vi "FGVData.vi"(7 "Enum":T1, 8 "error in":errorcluster, 9 "DataIn":sgl[](array[numeric])) -> (0 "error out":errorcluster, 1 "DataOut":sgl[](array[numeric]))   [LabVIEW 2016]
uses:
  controls/Enum.ctl
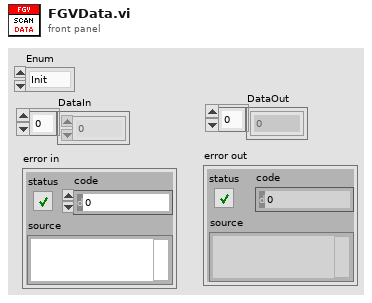
[diagram p1: front panel]
types:
  T1 = typedef "Enum.ctl" = enum16{"Init", "Read", "Write"}
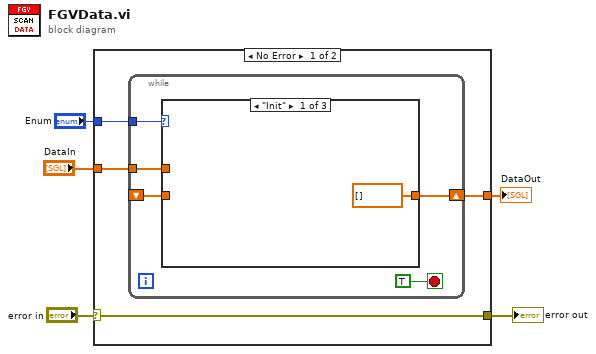
[diagram p0: block diagram]
diagram:
  n1 = case shown="No Error" "error in" {
    selector: "error in" -> [w8 w19]
    tunnel: "Enum" -> [w9 _]
    tunnel: [w8 w19] -> w4
    tunnel: "DataIn" -> [w7 w18]
    tunnel: [w6 w18] -> w1
    frame No Error {
      n2 = while {
        tunnel: w9 -> [w13]
        tunnel: w7 -> [w11]
        shift-right: [w12] -> w6
        shift-left: _ -> [w10]
        stop <- TRUE stop-if-true
        n3 = case shown="\"Init\"" w13 {
          tunnel: [sgl[] [] ("DataIn") w16 w17] -> w12
          tunnel: w11 -> [_ _ w17]
          tunnel: w10 -> [_ w16 _]
          frame "Init" {
          }
          frame "Read", Default {
          }
          frame "Write" {
          }
        }
      }
    }
    frame Error {
    }
  }
  "error out" <- w4
  "DataOut" <- w1
